vi "Configure Frequency Sweep.vi"(0 "VISA resource name":refnum<visa-resource-name>, 1 "Enable Frequency Sweep (T: Enable)":bool=TRUE, 5 "Channel (0: Channel 1)":u16(ring) items=["Channel 1", "Channel 2"], 7 "Sweep Spacing (0: Linear)":u16(ring) items=["Linear", "Log"], 9 "Sweep Time (1.00 s)":dbl=1.0 format="%#.6g", 11 "error in (no error)":errorcluster, 12 "Start Frequency (100 Hz)":dbl=100.0 format="%#.6g", 13 "Stop  Frequency  (1000 Hz)":dbl=1000.0 format="%#.6g") -> (4 "VISA resource name out":refnum<visa-resource-name>, 15 "error out":errorcluster)   [LabVIEW 2019, in "Tektronix AFG 3000 Series.lvlib"]
doc: "Configures and enables a frequency sweep. In the frequency sweep mode, the function generator steps from the start frequency to the stop frequency at a sweep rate."
uses:
  Tektronix AFG 3000 Series.lvlib
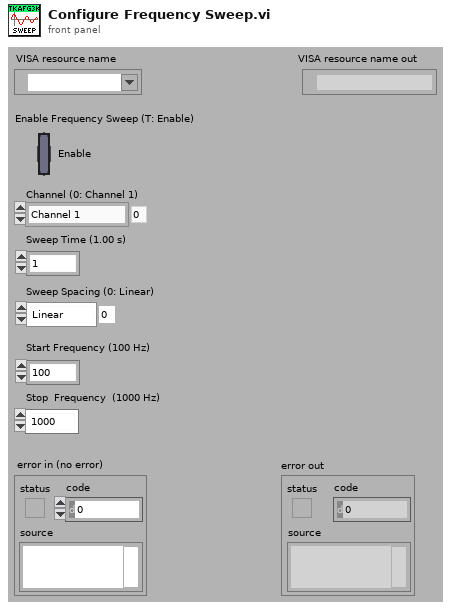
[diagram p1: front panel]
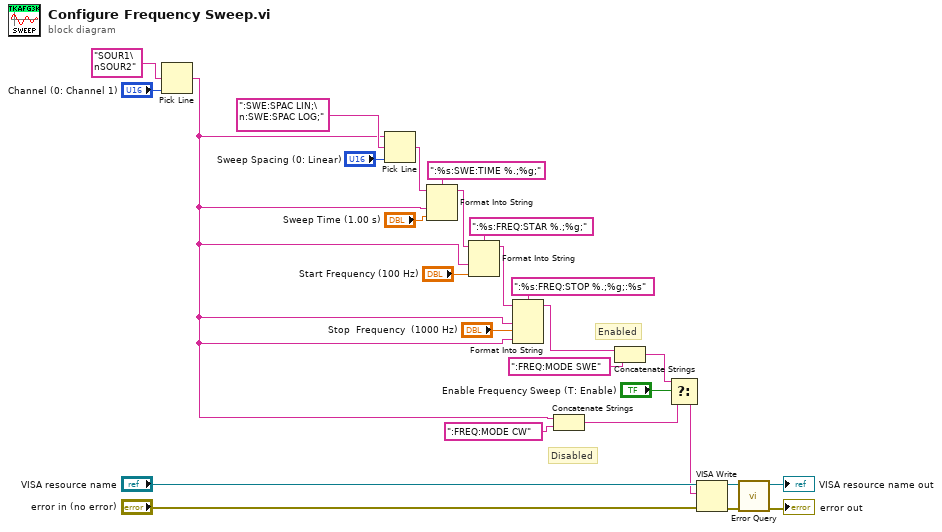
[diagram p0: block diagram]
diagram:
  # "Disabled"
  # "Enabled"
  n1 = Pick Line(multi-line string="SOUR1\nSOUR2" ("string (\"\")"), line index="Channel (0: Channel 1)") -> (output string=w1:string)  [unwired: 1 in]
  n2 = Pick Line(string ("")=w1, multi-line string=":SWE:SPAC LIN;\n:SWE:SPAC LOG;", line index="Sweep Spacing (0: Linear)") -> (output string=w5:string)
  n3 = Format Into String(format string=":%s:SWE:TIME %.;%g;", initial string=w5, w1, "Sweep Time (1.00 s)") -> (resulting string=w19:string)  [unwired: 1 in, 1 out]
  n4 = Format Into String(format string=":%s:FREQ:STAR %.;%g;", initial string=w19, w1, "Start Frequency (100 Hz)") -> (resulting string=w16:string)  [unwired: 1 in, 1 out]
  n5 = Format Into String(format string=":%s:FREQ:STOP %.;%g;:%s", initial string=w16, w1, "Stop  Frequency  (1000 Hz)", w1) -> (resulting string=w8:string)  [unwired: 1 in, 1 out]
  n6 = Concatenate Strings(w1, ":FREQ:MODE CW" ("Disable")) -> (w10:string)
  n7 = Concatenate Strings(w8, ":FREQ:MODE SWE" ("Enable")) -> (w12:string)
  n8 = Select(t=w12, s="Enable Frequency Sweep (T: Enable)", f=w10) -> (s? t:f=w9:string)
  n9 = VISA Write(VISA resource name="VISA resource name", write buffer=w9, error in (no error)="error in (no error)") -> (VISA resource name out=w25:refnum<visa-resource-name>, error out=w23:errorcluster)  [unwired: 1 out]
  n10 = call "Error Query.vi"("error in (no error)"=w23, "VISA resource name"=w25) -> ("error out"=→"error out":errorcluster, "VISA resource name out"=→"VISA resource name out":refnum<visa-resource-name>)  [unwired: 6 in, 2 out]
